vi "DFD FXP MRate Simulation (I32).vi"(5 "input range":dbl=1.0, 7 "init? (T)":bool=TRUE, 8 "error in (no error)":errorcluster, 10 "multirate filter":T1={"mMRate_Structure"=enum."IIR", "mMRate_Mode"=0, "mMRate_Factor"=-1, "mMRate_FIRParams"={"mMRate_FIR_H"=[], "mMRate_FIR_IsNyquist?"=FALSE, "mMRate_FIR_IsSymmetric?"=FALSE}, "mMRate_CICParams"={"mMRate_CIC_#Stage"=0, "mMRate_CIC_Lag"=0, "mMRate_CIC_Type"=enum."Lowpass"}, "mMRate_Order"=0, "mMRate_Version"="2.0", "mMRate_Comments"="", "mMRate_RationalFactor"={"mMRate_L"=-1, "mMRate_M"=-1}, "mMRate_Fs"=1.0, "mMRate_Quantized?"=FALSE, "mMRate_QFilterGain"=1.0, "mMRate_CoefWl"=16, "mMRate_Scaling"={"mMRate_ScaleByPowerOf2?"=FALSE, "mMRate_ScaleType"=enum."No Norm"}, "mMRate_InputWl"=16, "mMRate_OutputWl"=16, "mMRate_OutputMode"=enum."Truncation", "mMRate_MultMode"=enum."Truncated", "mMRate_BitPruning"=FALSE, "mMRate_GainWl"=16, "mMRate_OutputFwl"=0, "mMRate_SumIwl"=0, "mMRate_InputIwl "=16, "mMRate_SumWl"=32, "mMRate_CoefIwl"=0} {"mMRate_SumWl" min=1 max=32 step=1; "mMRate_InputIwl" min=1 max=32 step=1; "mMRate_GainWl" min=1 max=32 step=1; "mMRate_OutputWl" min=1 max=32 step=1; "mMRate_InputWl" min=1 max=32 step=1; "mMRate_CoefWl" min=1 max=32 step=1; "mMRate_Mode" items=["Default"=-1, "No Rate Change"=0, "Interpolation"=1, "Decimation"=2, "Interpolated"=3, "Rational"=4]}, 11 "signal in":i32[](array[numeric])) -> (0 "error out":errorcluster, 2 "integer signal out":i32[](array[numeric]), 3 "DBL signal out":dbl[](array[numeric]))   [LabVIEW 2017, in "NI_DigFilterLicensed.lvlib"]
doc: "Simulates the filtering process of a fixed-point multirate filter continuously. Wire data to the <B>signal in</B> input to determine the polymorphic instance to use or manually select the instance."
uses:
  <vilib>/addons/Digital Filter Design/NI_DigFilterLicensed.lvlib
  <vilib>/addons/Digital Filter Design/_Objects.llb/DFD Multirate Filter Obj.ctl
  <vilib>/addons/Digital Filter Design/_Objects.llb/DFD Multirate Mode.ctl
  <vilib>/addons/Digital Filter Design/_Objects.llb/DFD Coef Norm Type.ctl
  <vilib>/addons/Digital Filter Design/_Objects.llb/DFD Round-off Mode.ctl
  <vilib>/addons/Digital Filter Design/_Objects.llb/DFD FXP MRate Multiply Mode.ctl
  <vilib>/addons/Digital Filter Design/FXPMRateSim.llb/DFD FXP MRate Postprocessing (I32, 1Ch).vi
  <vilib>/addons/Digital Filter Design/NI_DigFilter_FXP.lvlib
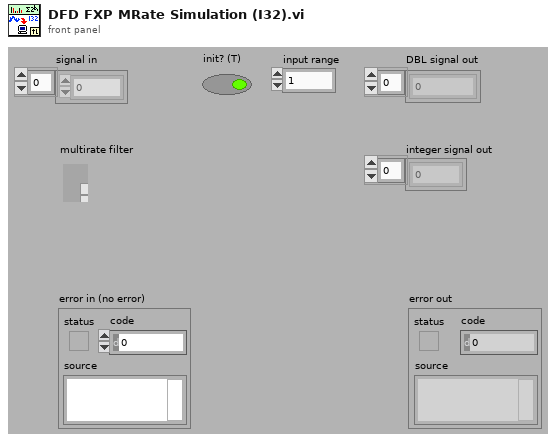
[diagram p1: front panel]
types:
  T1 = typedef "NI_DigFilterLicensed.lvlib/DFD Multirate Filter Obj.ctl" = cluster{"mMRate_Structure":enum16{"CIC", "FIR", "IIR", "Lattice"}, "mMRate_Mode":T2, "mMRate_Factor":i32, "mMRate_FIRParams":cluster{"mMRate_FIR_H":dbl[], "mMRate_FIR_IsNyquist?":bool, "mMRate_FIR_IsSymmetric?":bool}, "mMRate_CICParams":cluster{"mMRate_CIC_#Stage":i32, "mMRate_CIC_Lag":i32, "mMRate_CIC_Type":enum16{"Lowpass", "Highpass"}}, "mMRate_Order":i32, "mMRate_Version":string, "mMRate_Comments":string, "mMRate_RationalFactor":cluster{"mMRate_L":i32, "mMRate_M":i32}, "mMRate_Fs":dbl, "mMRate_Quantized?":bool, "mMRate_QFilterGain":dbl, "mMRate_CoefWl":i16, "mMRate_Scaling":cluster{"mMRate_ScaleByPowerOf2?":bool, "mMRate_ScaleType":T3}, "mMRate_InputWl":i16, "mMRate_OutputWl":i16, "mMRate_OutputMode":T4, "mMRate_MultMode":T5, "mMRate_BitPruning":bool, "mMRate_GainWl":i16, "mMRate_OutputFwl":i16, "mMRate_SumIwl":i16, "mMRate_InputIwl ":i16, "mMRate_SumWl":i16, "mMRate_CoefIwl":i16}
  T2 = typedef "NI_DigFilterLicensed.lvlib/DFD Multirate Mode.ctl" = i16
  T3 = typedef "NI_DigFilterLicensed.lvlib/DFD Coef Norm Type.ctl" = enum16{"No Norm", "Time Domain 1-Norm", "Time Domain 2-Norm", "Time Domain Inf-Norm"}
  T4 = typedef "NI_DigFilterLicensed.lvlib/DFD Round-off Mode.ctl" = enum16{"Nearest", "Truncation"}
  T5 = typedef "NI_DigFilterLicensed.lvlib/DFD FXP MRate Multiply Mode.ctl" = enum16{"Truncated", "Full"}
  T6 = typedef "dfd_FXP MRate Simu State.ctl" = cluster{"acc1":T7[], "acc2":T7[], "FIR state":i64[], "next phase":i32}
  T7 = typedef "dfd_Integer I160.ctl" = cluster{"Hi [I32]":i32, "Lo3 [U32]":u32, "Lo2 [U32]":u32, "Lo1 [U32]":u32, "Lo0 [U32]":u32}
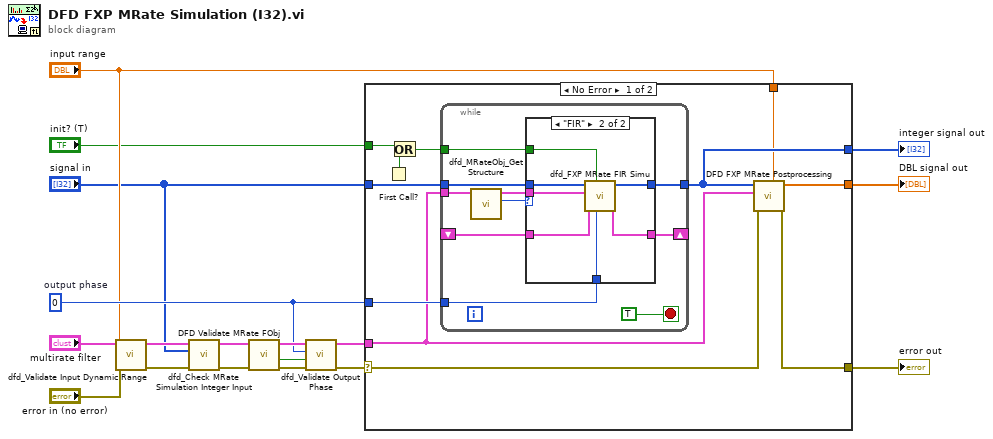
[diagram p0: block diagram]
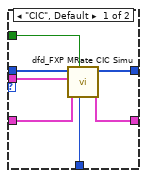
[diagram p2: hidden frame]
diagram:
  w13 = 0  # output phase
  n1 = call <vilib>:"dfd_Validate Input Dynamic Range.vi"("error in (no error)"="error in (no error)", "input range"="input range") -> ("error out"=w6:errorcluster)  [unwired: 9 out]
  n2 = call <vilib>:"dfd_Check MRate Simulation Integer Input.vi"("error in (no error)"=w6, "signal in"="signal in", "multirate filter"="multirate filter") -> ("error out"=w5:errorcluster, "dup multirate filter"=w3:T1)  [unwired: 7 out]
  n3 = call <vilib>:"DFD Validate MRate FObj.vi"("error in (no error)"=w5, "multirate filter in"=w3) -> ("error out"=w14:errorcluster, "is valid FXP?"=w12:bool, "multirate filter out"=w15:T1)  [unwired: 7 out]
  n4 = call <vilib>:"dfd_Validate Output Phase.vi"("error in (no error)"=w14, "is valid FXP?"=w12, "output phase"=w13, "multirate filter in"=w15) -> ("error out"=w7:errorcluster, "dup multirate filter"=w8:T1)  [unwired: 6 out]
  n5 = case shown="No Error" w7 {
    selector: w7 -> [w24 w53]
    tunnel: "signal in" -> [w28 _]
    tunnel: "input range" -> [w22 _]
    tunnel: [w27 _] -> w17
    tunnel: w8 -> [w18 _]
    tunnel: [w26 w53] -> w16
    tunnel: w13 -> [w25 _]
    tunnel: [w23 _] -> w9
    tunnel: "init? (T)" -> [w21 _]
    frame No Error {
      n6 = First Call?() -> (First Call?: T/F=w20:bool)
      n7 = Or(x=w21, y=w20) -> (x .or. y?=w19:bool)
      n8 = while {
        tunnel: w28 -> [w38]
        tunnel: w18 -> [w35]
        tunnel: w25 -> [w34]
        tunnel: [w33] -> w23
        shift-right: [w31] -> _
        shift-left: _ -> [w30]
        tunnel: w19 -> [w29]
        stop <- TRUE stop-if-true
        n9 = call <vilib>:"dfd_MRateObj_Get Structure.vi"("multirate filter in"=w35) -> ("structure"=w37:enum16{"CIC", "FIR", "IIR", "Lattice"}, "dup multirate filter"=w36:T1)  [unwired: 9 out]
        n10 = case shown="\"FIR\"" w37 {
          tunnel: w36 -> [w42 w49]
          tunnel: w38 -> [w44 w52]
          tunnel: w34 -> [w45 w50]
          tunnel: [w43 w51] -> w33
          tunnel: w29 -> [w41 w48]
          tunnel: [w40 w46] -> w31
          tunnel: w30 -> [w39 w47]
          frame "CIC", Default {
            n11 = call <vilib>:"dfd_FXP MRate CIC Simu.vi"("output phase"=w45, "init? (T)"=w41, "FXPMRateSimState in"=w39, "FXP CIC"=w42, "signal in"=w44) -> ("FXPMRateSimState out"=w40:T6, "signal out"=w43:i32[])  [unwired: 1 in, 4 out]
          }
          frame "FIR" {
            n12 = call <vilib>:"dfd_FXP MRate FIR Simu.vi"("output phase"=w50, "init? (T)"=w48, "FXPMRateSimState in"=w47, "multirate filter"=w49, "signal in"=w52) -> ("FXPMRateSimState out"=w46:T6, "signal out"=w51:i32[])  [unwired: 5 out]
          }
        }
      }
      n13 = call-poly <vilib>:"DFD FXP MRate Postprocessing.vi"("input range"=w22, "error in (no error)"=w24, "multirate filter"=w18, "signal in"=w23) -> ("error out"=w26:errorcluster, "signal out"=w27:dbl[])  [unwired: 1 in, 5 out]
    }
    frame Error {
    }
  }
  "error out" <- w16
  "DBL signal out" <- w17
  "integer signal out" <- w9
